vi "1.3.1-ParseYPR.vi"(10 "Serial Byte":u8) -> (1 "Yaw":fxp<+/-,64,32> format="%.42g", 2 "Heading (out)":T1)   [LabVIEW 2010]
doc: "This VI parses Yaw, Pitch, and Roll (YPR) data from the VectorNav. In response to a YPR Read Request, the VectorNav will reply in the form \"$VNYPR,XX,-XXX.XX,-XXX.XX,+XXX.XX*XX\" (where X is a digit from 0-9). This string is in the form \"$<command type>,<access ID>, <yaw>,<pitch>,<roll>\".\n\nThe VI first waits for a $, then checks to make sure it has read \"VNYPR,\" correctly, then adds up each of the XX values and saves them appropriately. Since it receives these values one byte at a time , it must do some simple fixed point math to make sure the appropriate decimal value is saved."
uses:
  1.3.1-ParseYPR.ctl
panel:
  in  "Heading (in)":T1 {"Yaw" format="%.42g"; "Pitch" format="%.42g"; "Roll" format="%.42g"}
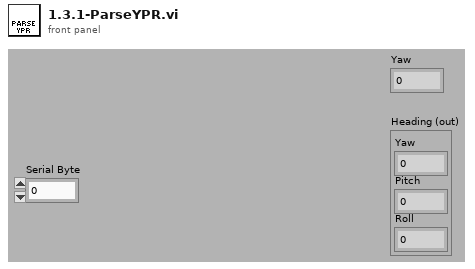
[diagram p1: front panel]
types:
  T1 = cluster{"Yaw":fxp<+/-,64,32>, "Pitch":fxp<+/-,64,32>, "Roll":fxp<+/-,64,32>}
  T2 = typedef "1.3.1-ParseYPR.ctl" = enum16{"Wait for $", "Check VNYPR", "Read numbers"}
  T3 = enum16{"Initialize", "Yaw", "Pitch", "Roll", "Done"}
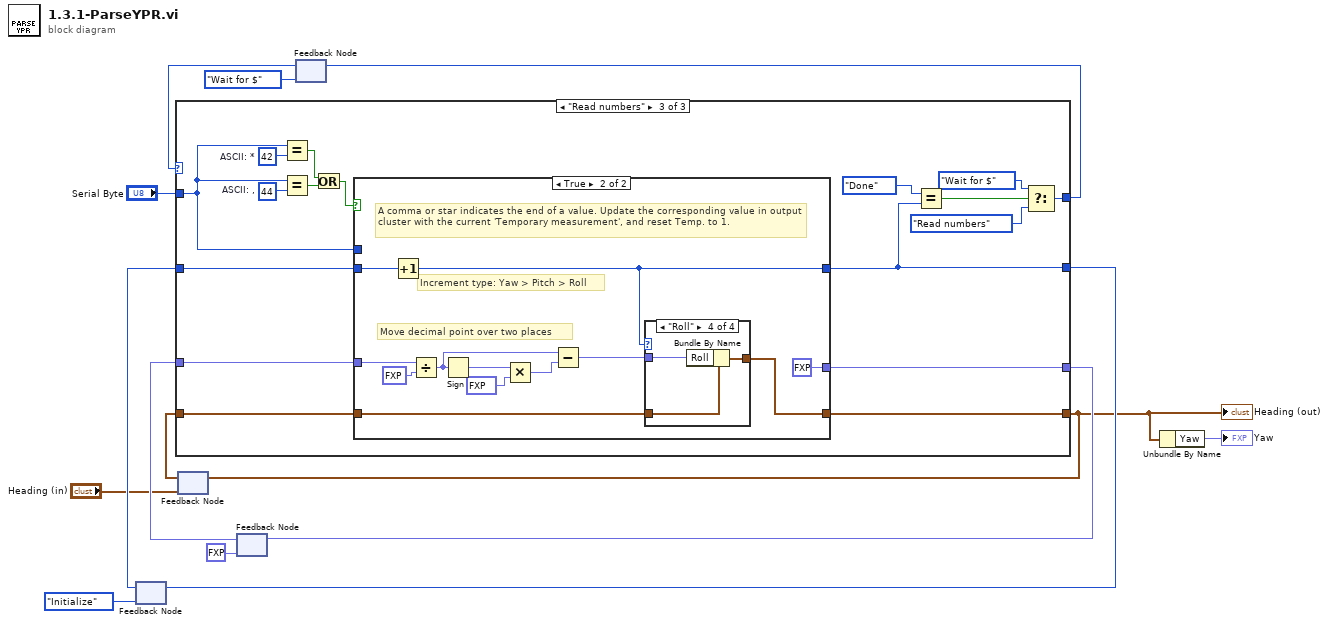
[diagram p0: block diagram]
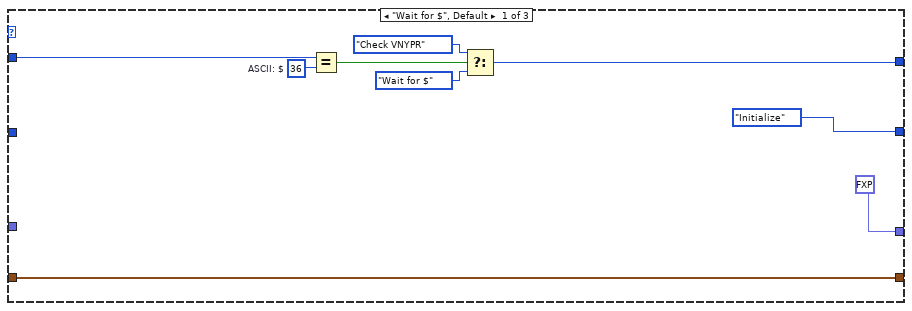
[diagram p2: hidden frame]
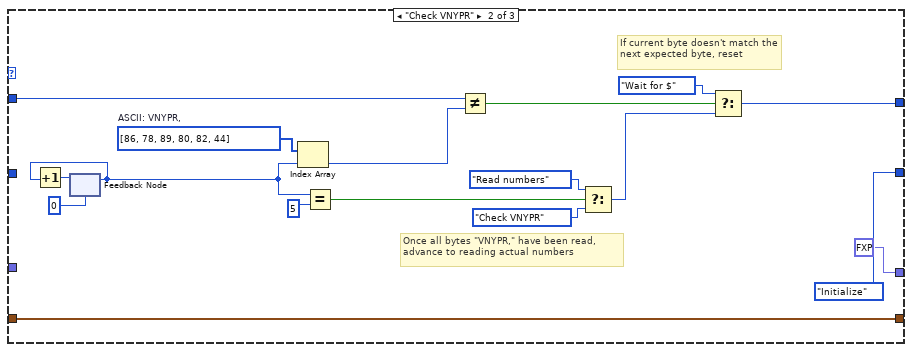
[diagram p3: hidden frame]
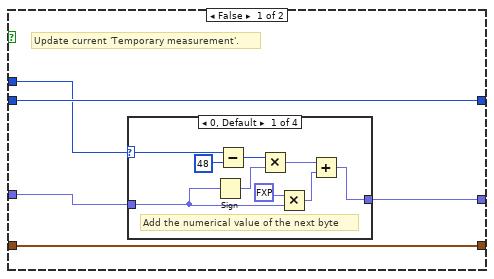
[diagram p4: hidden frame]
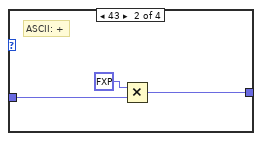
[diagram p5: hidden frame]
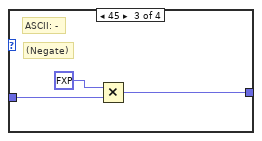
[diagram p6: hidden frame]
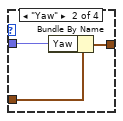
[diagram p9: hidden frame]
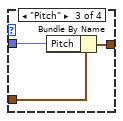
[diagram p10: hidden frame]
diagram:
  n1 = feedback #1(T3."Initialize" ("f")) -> (w6:T3)
  n2 = feedback #2("Heading (in)") -> (w9:T1)
  n3 = feedback #3(fxp<+/-,64,32> 1.0 ("Yaw")) -> (w11:fxp<+/-,64,2047>)
  n4 = feedback #4(1.3.1-ParseYPR."Wait for $" ("1.3.1-ParseYPR")) -> (w12:T2)
  n5 = case shown="\"Read numbers\"" w12 {
    tunnel: [w20 w29 w44] -> w14
    tunnel: "Serial Byte" -> [w23 w36 w43]
    tunnel: w11 -> [_ _ w45]
    tunnel: [fxp<+/-,32,12> 1.0 ("Yaw") fxp<+/-,32,12> 1.0 ("Yaw") w46] -> w5
    tunnel: [w19 w37 w55] -> w1
    tunnel: w9 -> [w19 w37 w56]
    tunnel: [T3."Initialize" ("f") T3."Initialize" ("f") w53] -> w7
    tunnel: w6 -> [_ _ w54]
    frame "Wait for $", Default {
      w22 = u8 36  # ASCII: $
      n6 = Equal?(x=w23, y=w22) -> (x = y?=w21:bool)
      n7 = Select(t=1.3.1-ParseYPR."Check VNYPR" ("1.3.1-ParseYPR"), s=w21, f=1.3.1-ParseYPR."Wait for $" ("1.3.1-ParseYPR")) -> (s? t:f=w20:T2)
    }
    frame "Check VNYPR" {
      w40 = u8[] [86, 78, 89, 80, 82, 44]  # ASCII: VNYPR,
      # "If current byte doesn't match the next expected byte, reset"
      # "Once all bytes \"VNYPR,\" have been read, advance to reading actual numbers"
      n8 = feedback #5(0 ("Serial Byte")) -> (w24:i32)
      n9 = Increment(x=w24) -> (x+1=w25:i32)
      n10 = feedback-in #5(w25) -> ()
      n11 = Index Array(array=w40, index=w24) -> (element=w39:u8)
      n12 = Equal?(x=w24, y=5) -> (x = y?=w34:bool)
      n13 = Not Equal?(x=w36, y=w39) -> (x != y?=w38:bool)
      n14 = Select(t=1.3.1-ParseYPR."Read numbers" ("1.3.1-ParseYPR"), s=w34, f=1.3.1-ParseYPR."Check VNYPR" ("1.3.1-ParseYPR")) -> (s? t:f=w27:T2)
      n15 = Select(t=1.3.1-ParseYPR."Wait for $" ("1.3.1-ParseYPR"), s=w38, f=w27) -> (s? t:f=w29:T2)
    }
    frame "Read numbers" {
      w50 = u8 42  # ASCII: *
      w57 = u8 44  # ASCII: ,
      n16 = Equal?(x=w43, y=w50) -> (x = y?=w48:bool)
      n17 = Equal?(x=w43, y=w57) -> (x = y?=w49:bool)
      n18 = Or(x=w48, y=w49) -> (x .or. y?=w47:bool)
      n19 = case shown="True" w47 {
        tunnel: w56 -> [w62 w90]
        tunnel: [w62 w89] -> w55
        tunnel: [w61 w87] -> w53
        tunnel: w54 -> [w61 w88]
        tunnel: [w58 fxp<+/-,32,12> 1.0 ("Yaw")] -> w46
        tunnel: w45 -> [w59 w86]
        tunnel: w43 -> [w60 _]
        frame False {
          # "Update current 'Temporary measurement'."
          n20 = case shown="0, Default" w60 {
            selector: w60 -> [w69 _ _ _]
            tunnel: w59 -> [w70 w74 w77 w78]
            tunnel: [w64 w73 w76 w78] -> w58
            frame 0, Default {
              # "Add the numerical value of the next byte"
              n21 = Sign(1:w70) -> (0:w66:fxp<+/-,2,2>)
              n22 = Subtract(x=w69, y=u8 48) -> (x-y=w67:u8)
              n23 = Multiply(x=w67, y=w66) -> (x*y=w65:fxp<+/-,9,9>)
              n24 = Multiply(x=fxp<+/-,32,12> 10.0 ("Yaw"), y=w70) -> (x*y=w71:fxp)
              n25 = Add(x=w65, y=w71) -> (x+y=w64:fxp)
            }
            frame 43 {
              # "ASCII: +"
              n26 = Multiply(x=fxp<+/-,32,12> 1.0 ("Yaw"), y=w74) -> (x*y=w73:fxp)
            }
            frame 45 {
              # "(Negate)"
              # "ASCII: -"
              n27 = Multiply(x=fxp<+/-,32,12> -1.0 ("Yaw"), y=w77) -> (x*y=w76:fxp)
            }
            frame 46 {
              # "(Ignore decimal for now)"
              # "ASCII: ."
            }
          }
        }
        frame True {
          # "Increment type: Yaw > Pitch > Roll"
          # "Move decimal point over two places"
          # "A comma or star indicates the end of a value. Update the corresponding value in output cluster with the current 'Temporary measurement', and reset Temp. to 1."
          n28 = Increment(x=w88) -> (x+1=w87:T3)
          n29 = Divide(x=w86, y=fxp<+/-,32,12> 100.0 ("Yaw")) -> (x/y=w84:fxp)
          n30 = Sign(1:w84) -> (0:w82:fxp<+/-,2,2>)
          n31 = Multiply(x=w82, y=fxp<+/-,32,12> 1000.0 ("Yaw")) -> (x*y=w83:fxp<+/-,33,13>)
          n32 = Subtract(x=w84, y=w83) -> (x-y=w85:fxp)
          n33 = case shown="\"Roll\"" w87 {
            tunnel: [w91 w94 w97 w100] -> w89
            tunnel: w90 -> [w91 w93 w96 w99]
            tunnel: w85 -> [_ w92 w95 w98]
            frame "Initialize", Default {
            }
            frame "Yaw" {
              n34 = Bundle By Name(cluster=w93, "Yaw"=w92) -> (w94:T1)
            }
            frame "Pitch" {
              n35 = Bundle By Name(cluster=w96, "Pitch"=w95) -> (w97:T1)
            }
            frame "Roll" {
              n36 = Bundle By Name(cluster=w99, "Roll"=w98) -> (w100:T1)
            }
          }
        }
      }
      n37 = Equal?(x=T3."Done", y=w53) -> (x = y?=w51:bool)
      n38 = Select(t=1.3.1-ParseYPR."Wait for $" ("1.3.1-ParseYPR"), s=w51, f=1.3.1-ParseYPR."Read numbers" ("1.3.1-ParseYPR")) -> (s? t:f=w44:T2)
    }
  }
  "Heading (out)" <- w1
  n39 = feedback-in #1(w7) -> ()
  n40 = feedback-in #2(w1) -> ()
  n41 = feedback-in #3(w5) -> ()
  n42 = feedback-in #4(w14) -> ()
  n43 = Unbundle By Name(w1) -> ("Yaw"=→"Yaw":fxp<+/-,64,32>)
